vi "ActionVIOnCompile.vi"(8 "error in (no error)":errorcluster, 11 "Device Item Ref in":T1 format="%.0x") -> (0 "error out":errorcluster)   [LabVIEW 2019, in "FPGA Addon System Explorer.lvlib"]
uses:
  FPGA Addon System Explorer.lvlib
  <vilib>/NI VeriStand/Custom Device API/Custom Device API.lvlib
  <vilib>/NI VeriStand/Custom Device API/Data Access Type.ctl
  Addon Shared/Constants.vi
  Addon Shared/FPGA Addon Shared.lvlib
  Addon Shared/FG Action.ctl
  Addon Shared/Delacing Scheme.ctl
  Addon Shared/DMA Settings.ctl
  <vilib>/NI VeriStand/Custom Device API/Data Reference.ctl
  Addon Shared/Compiled.DMASettings.ctl
  <vilib>/NI VeriStand/Custom Device API/Block Data Reference.ctl
  Addon Shared/Scalar Type.ctl
  <vilib>/NI VeriStand/Custom Device API/Waveform Data Reference.ctl
  Addon Shared/Compiled.Settings.ctl
  Addon Shared/Register Information.ctl
  Addon Shared/Compiled.RegisterSettings.ctl
  Addon Shared/FPGA Settings.ctl
  Addon Shared/DMA Acquisition Mode.ctl
  <vilib>/NI/NIVS Inline Async API/_Data Access System Explorer/Data Access System Explorer.lvlib
  <vilib>/NI VeriStand/Custom Device API/Custom Device Target Type.ctl
  <vilib>/NI VeriStand/Custom Device API/Set Item Property (Variant).vi
  <vilib>/NI VeriStand/Custom Device Tools/Custom Device Utility Library/Custom Device Utility Library.lvlib
  Addon Shared/Data Type.ctl
  <vilib>/NI VeriStand/Custom Device API/Custom Device Item Ref.ctl
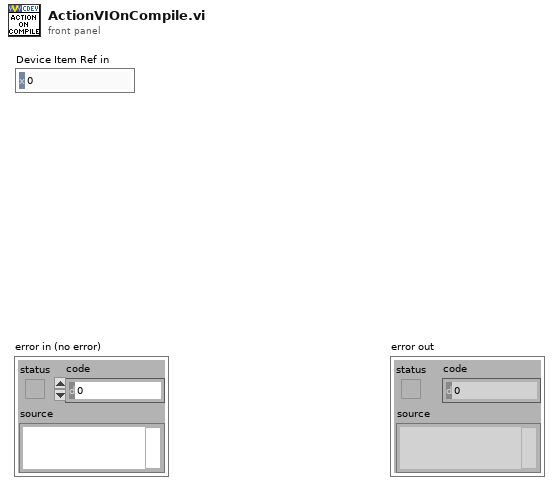
[diagram p1: front panel]
types:
  T1 = typedef "Custom Device API.lvlib/Custom Device Item Ref.ctl" = u64
  T2 = typedef "FPGA Addon Shared.lvlib/Compiled.Settings.ctl" = cluster{"Name":string, "IncomingRegisters.Settings":T3[], "IncomingRegisters.Refs":cluster{"Refs":T7[], "Values":dbl[]}, "OutgoingRegisters.Settings":T3[], "OutgoingRegisters.Refs":cluster{"Refs":T7[], "Values":dbl[]}, "Incoming.Size":i32, "Outgoing.Size":i32, "IncomingDMA.Settings":T9[], "OutgoingDMA.Settings":T9[], "FPGA.Settings":T14, "Target.Type":T15}
  T3 = typedef "FPGA Addon Shared.lvlib/Compiled.RegisterSettings.ctl" = cluster{"Scalar Type":T4, "Index":i32, "Length":i32, "Register":T5}
  T4 = typedef "FPGA Addon Shared.lvlib/Scalar Type.ctl" = enum16{"Standard", "Bitpacked"}
  T5 = typedef "FPGA Addon Shared.lvlib/Register Information.ctl" = cluster{"Name":string, "Data Type":T6, "Default Value":variant}
  T6 = typedef "FPGA Addon Shared.lvlib/Data Type.ctl" = enum8{"<Null>", "I8", "I16", "I32", "I64", "U8", "U16", "U32", "U64", "SGL", "Boolean", "Analog PWM In Settings", "Analog PWM In", "Digital PWM In Settings", "Digital PWM In", "Digital PWM Out", "Sine Out", "FXP+/-24.5", "FXP+/-16.5", "FXP+/-32.8", "FXP+/-64.32", "FXP+/-16.7", "FXP+/-20.5", "FXP+/-27.5", "FXP+/-32.16", "FXP +16.3", "FXP +18.3", "Digital Static In", "Digital Static Out", "Digital Static In Settings", "Digital WSS Out", "Quad Encoder Settings", "Quad Encoder In"}
  T7 = typedef "Custom Device API.lvlib/Block Data Reference.ctl" = cluster{"Data Reference":T8, "Offset":u64, "Length":u64}
  T8 = typedef "Custom Device API.lvlib/Data Reference.ctl" = i32
  T9 = typedef "FPGA Addon Shared.lvlib/Compiled.DMASettings.ctl" = cluster{"Name":string, "Data Type":T6, "DMA.Settings":T10, "DMA.VSRefs":T13[]}
  T10 = typedef "FPGA Addon Shared.lvlib/DMA Settings.ctl" = cluster{"Number of Channels":u8, "Delacing Scheme":T11, "Update Rate":u32, "dt":dbl, "Mode":T12, "Number of Samples":u32, "DMA Host Buffer":u32}
  T11 = typedef "FPGA Addon Shared.lvlib/Delacing Scheme.ctl" = enum8{"Interleaved", "Bitpacked"}
  T12 = typedef "FPGA Addon Shared.lvlib/DMA Acquisition Mode.ctl" = enum8{"Continuous", "Triggered Finite"}
  T13 = typedef "Custom Device API.lvlib/Waveform Data Reference.ctl" = i32
  T14 = typedef "FPGA Addon Shared.lvlib/FPGA Settings.ctl" = cluster{"Bitfile path":path, "RIO Device Address":string}
  T15 = typedef "Custom Device API.lvlib/Custom Device Target Type.ctl" = enum16{"PharLap", "VxWorks", "Windows", "Linux_32_ARM", "Linux_x64"}
  T16 = typedef "Custom Device API.lvlib/Data Access Type.ctl" = enum16{"Read", "Write"}
  T17 = typedef "FPGA Addon Shared.lvlib/FG Action.ctl" = enum8{"GET", "SET"}
  T18 = typedef "Custom Device API.lvlib/Custom Device Item Info.ctl" = cluster{"Name":string, "Is Channel":bool, "GUID":string, "Is Waveform":bool}
  T19 = cluster{"Name":string, "Type":enum16{"Output/Write", "Input/Read", "Input/ReadWrite"}, "VS Refs":T1[]}[]
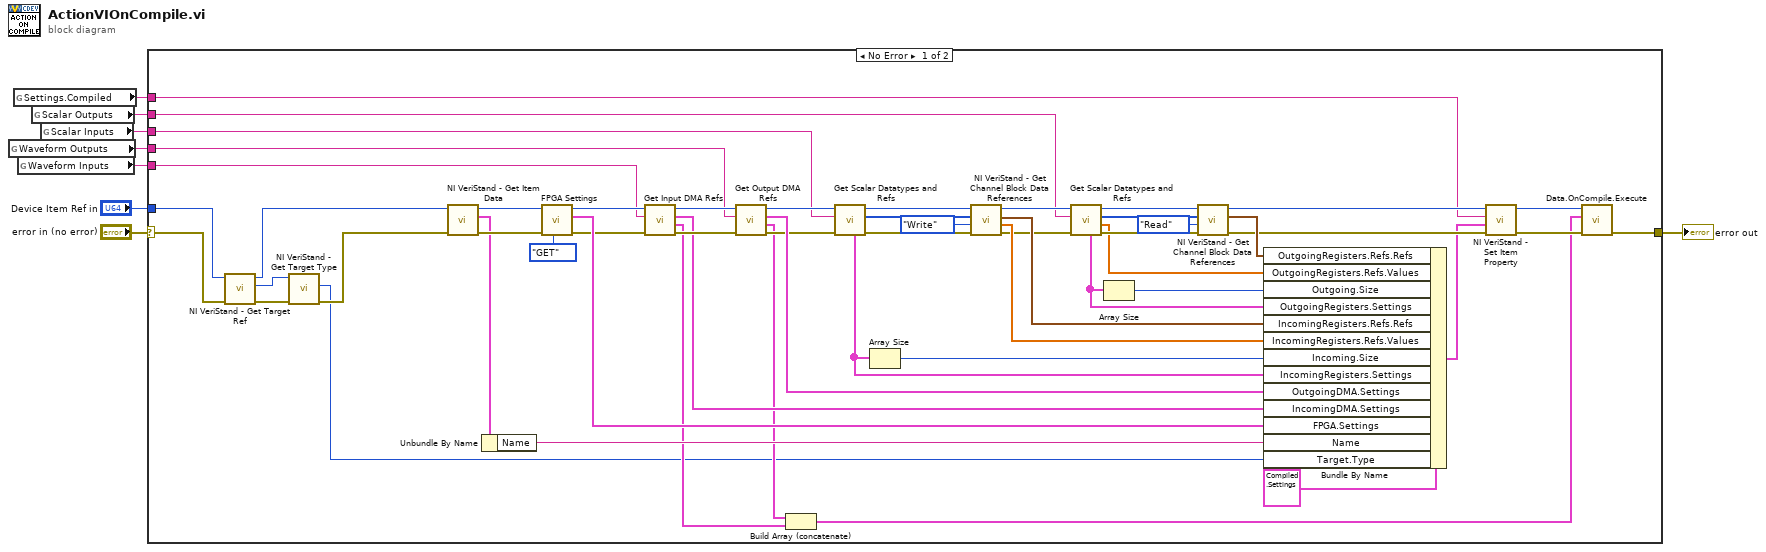
[diagram p0: block diagram]
diagram:
  n1 = global read "Constants.vi" "Waveform Outputs"() -> (w4:string)
  n2 = global read "Constants.vi" "Settings.Compiled"() -> (w1:string)
  n3 = global read "Constants.vi" "Waveform Inputs"() -> (w5:string)
  n4 = global read "Constants.vi" "Scalar Outputs"() -> (w2:string)
  n5 = global read "Constants.vi" "Scalar Inputs"() -> (w3:string)
  n6 = case shown="No Error" "error in (no error)" {
    selector: "error in (no error)" -> [w14 w63]
    tunnel: [w19 w63] -> w7
    tunnel: "Device Item Ref in" -> [w12 _]
    tunnel: w5 -> [w29 _]
    tunnel: w4 -> [w28 _]
    tunnel: w3 -> [w27 _]
    tunnel: w2 -> [w26 _]
    tunnel: w1 -> [w23 _]
    frame No Error {
      n7 = call <vilib>:"NI VeriStand - Get Target Ref.vi"("error in"=w14, "Item Ref in"=w12) -> ("error out"=w16:errorcluster, "Target Ref"=w15:T1, "Item Ref out"=w11:T1)  [unwired: 6 in, 1 out]
      n8 = call <vilib>:"NI VeriStand - Get Target Type.vi"("error in (no error)"=w16, "Item Ref in"=w15) -> ("error out"=w13:errorcluster, "Target Type"=w10:T15)  [unwired: 7 in, 1 out]
      n9 = call <vilib>:"NI VeriStand - Get Item Data.vi"("error in (no error)"=w13, "Item Ref in"=w11) -> ("error out"=w60:errorcluster, "Item Info"=w48:T18, "Item Ref out"=w59:T1)  [unwired: 6 in, 1 out]
      n10 = Unbundle By Name(w48) -> ("Name"=w49:string)
      n11 = call "FPGA Settings.vi"("Action"=FG_Action."GET", "error in (no error)"=w60, "Item Ref"=w59) -> ("error out"=w61:errorcluster, "FPGA Settings"=w62:T14, "Item Ref out"=w50:T1)  [unwired: 6 in]
      n12 = call "Get Input DMA Refs.vi"("error in (no error)"=w61, "Item GUID"=w29, "Section Ref in"=w50) -> ("error out"=w52:errorcluster, "Refs"=w22:T19, "DMA Settings"=w51:T9[], "Section Ref out"=w54:T1)  [unwired: 5 in]
      n13 = call "Get Output DMA Refs.vi"("error in (no error)"=w52, "Item GUID"=w28, "Section Ref in"=w54) -> ("error out"=w53:errorcluster, "Refs"=w21:T19, "DMA"=w56:T9[], "Section Ref out"=w55:T1)  [unwired: 5 in]
      n14 = Build Array (concatenate)(w21, w22) -> (w17:T19)
      n15 = call "Get Scalar Datatypes and Refs.vi"("error in (no error)"=w53, "Item GUID"=w27, "Section Ref in"=w55) -> ("error out"=w34:errorcluster, "VS Ref"=w32:T1[], "Section Ref out"=w33:T1, "Registers Ref"=w57:T3[])  [unwired: 4 in, 1 out]
      n16 = Array Size(array=w57) -> (size(s)=w46:i32)
      n17 = call <vilib>:"NI VeriStand - Get Channel Block Data References.vi"("error in (no error)"=w34, "Access"=Data_Access_Type."Write", "Channel Refs"=w32, "Device Ref in"=w33) -> ("error out"=w35:errorcluster, "Values Array"=w47:dbl[], "Block Data Refs"=w43:T7[], "Device Ref out"=w36:T1)  [unwired: 4 in]
      n18 = call "Get Scalar Datatypes and Refs.vi"("error in (no error)"=w35, "Item GUID"=w26, "Section Ref in"=w36) -> ("error out"=w38:errorcluster, "Default Values"=w9:dbl[], "VS Ref"=w40:T1[], "Section Ref out"=w39:T1, "Registers Ref"=w58:T3[])  [unwired: 4 in]
      n19 = Array Size(array=w58) -> (size(s)=w45:i32)
      n20 = call <vilib>:"NI VeriStand - Get Channel Block Data References.vi"("error in (no error)"=w38, "Access"=Data_Access_Type."Read", "Channel Refs"=w40, "Device Ref in"=w39) -> ("error out"=w30:errorcluster, "Block Data Refs"=w44:T7[], "Device Ref out"=w24:T1)  [unwired: 4 in, 1 out]
      n21 = Bundle By Name(cluster=T2 {"Name"="", "IncomingRegisters.Settings"=[], "IncomingRegisters.Refs"={"Refs"=[], "Values"=[]}, "OutgoingRegisters.Settings"=[], "OutgoingRegisters.Refs"={"Refs"=[], "Values"=[]}, "Incoming.Size"=0, "Outgoing.Size"=0, "IncomingDMA.Settings"=[], "OutgoingDMA.Settings"=[], "FPGA.Settings"={"Bitfile path"=path "", "RIO Device Address"=""}, "Target.Type"=enum."PharLap"}, "OutgoingRegisters.Refs.Refs"=w44, "OutgoingRegisters.Refs.Values"=w9, "Outgoing.Size"=w45, "OutgoingRegisters.Settings"=w58, "IncomingRegisters.Refs.Refs"=w43, "IncomingRegisters.Refs.Values"=w47, "Incoming.Size"=w46, "IncomingRegisters.Settings"=w57, "OutgoingDMA.Settings"=w56, "IncomingDMA.Settings"=w51, "FPGA.Settings"=w62, "Name"=w49, "Target.Type"=w10) -> (w25:T2)
      n22 = call-poly <vilib>:"NI VeriStand - Set Item Property.vi"("error in (no error)"=w30, "Value"=w25, "Property Name"=w23, "Item Ref in"=w24) -> ("error out"=w20:errorcluster, "Item Ref out"=w18:T1)  [unwired: 5 in, 1 out]
      n23 = call <vilib>:"Data.OnCompile.Execute.vi"("error in"=w20, "VS Ref Groups"=w17, "Custom Device Ref"=w18) -> ("error out"=w19:errorcluster)  [unwired: 7 in, 1 out]
    }
    frame Error {
    }
  }
  "error out" <- w7
